vi "cp.vi"(5 "DLLPath":path, 6 "error in (no error)":errorcluster, 7 "CP Parameters":T2={"Steps"=[{"vs_initial"=FALSE, "Current_step"=0.0, "Duration_step"=1.0}, {"vs_initial"=FALSE, "Current_step"=0.001, "Duration_step"=1.0}, {"vs_initial"=FALSE, "Current_step"=0.005, "Duration_step"=1.0}], "Step_number"=2, "N_Cycles"=0, "Record_every_dE"=0.005, "Record_every_dT"=0.05, "I_Range"=8, "E_Range"=3, "Bandwidth"=5, "em"=1, "ce"=0, "tb"=2.5e-05} {"tb" min=2.5e-05 max=1 format="%^_3e"; "ce" items=["Standard", "CE to ground"]; "N_Cycles" min=0 max=1000000; "Step_number" min=0 max=99; "E_Range" items=["±2.5V", "±5V", "±10V", "Auto"]; "Bandwidth" items=["1"=1, "2"=2, "3"=3, "4"=4, "5"=5, "6"=6, "7"=7, "8"=8, "9"=9]; "Record_every_dT" min=0.0001 max=1000 format="%^_3e"; "Record_every_dE" format="%^_3e"; "I_Range" items=["1pA", "1nA", "10nA", "100nA", "1µA", "10µA", "100µA", "1mA", "10mA", "100mA", "1A", "Booster"]; "Steps"."Duration_step" min=0.001 max=80000 format="%^_3e"; "Steps"."Current_step" min=-150 max=150 format="%^_3e"}, 8 "Channel":u8(ring) items=["1", "2", "3", "4", "5", "6", "7", "8", "9", "10", "11", "12", "13", "14", "15", "16"], 9 "IP adress":string="192.109.209.229") -> (0 "error out":errorcluster, 1 "XY Graph":cluster{"Data 101":sgl[], "Data 101":sgl[]}(graph), 2 "output cluster":T1, 3 "Exit 2":bool=TRUE)   [LabVIEW 2022 SP3]
doc: "The Chrono-Potentiometry (CP) is a controlled current technique. The current is controlled and the potential is the variable determined as a function of time.\nIn general, in this VI, the first thing to do is to start by establishing the connection with the instrument defined by its IP adress, then load the firmware in the channel selected, get the information on the plugged channels, load protocol on a channel, start/stop the protocol, retreive data and draw the graph."
uses:
  Library/EClib Functions/CPParameters.ctl
  Library/EClib Functions/Parameters.ctl
  Library/EClib Functions/EClib functions.lvlib
panel:
  out "cycle index":i32[](array[numeric])
  in  "Display Parameters?":bool caption="Display Parameters"
  out "DllPath":path caption="DLL Path"
  out "LibVersion":string caption="DLL Version"
  in  "Draw":enum16{"Ewe(t)", "I(t)"}(ring)
  out "Number of points":i32=5992
  out "Data 102":sgl[][](array[numeric]) format="%.2f"
  in  "stop":bool
  in  "Exit":bool
  in  "Start":bool
  # "Instructions:\nBefore running the VI you must type a valid IP adress that corresponds to the instrument.Then press the Run button to execute this VI.\nWhile this VI is running, choose the available channel, enter the CP parameters or keep the default values, then press the start button to begin the experience.\nChoose the waveform to draw (Ewe(t) or I(t)). You can stop the measure if you press the stop button and exit the execution if you press the exit button."
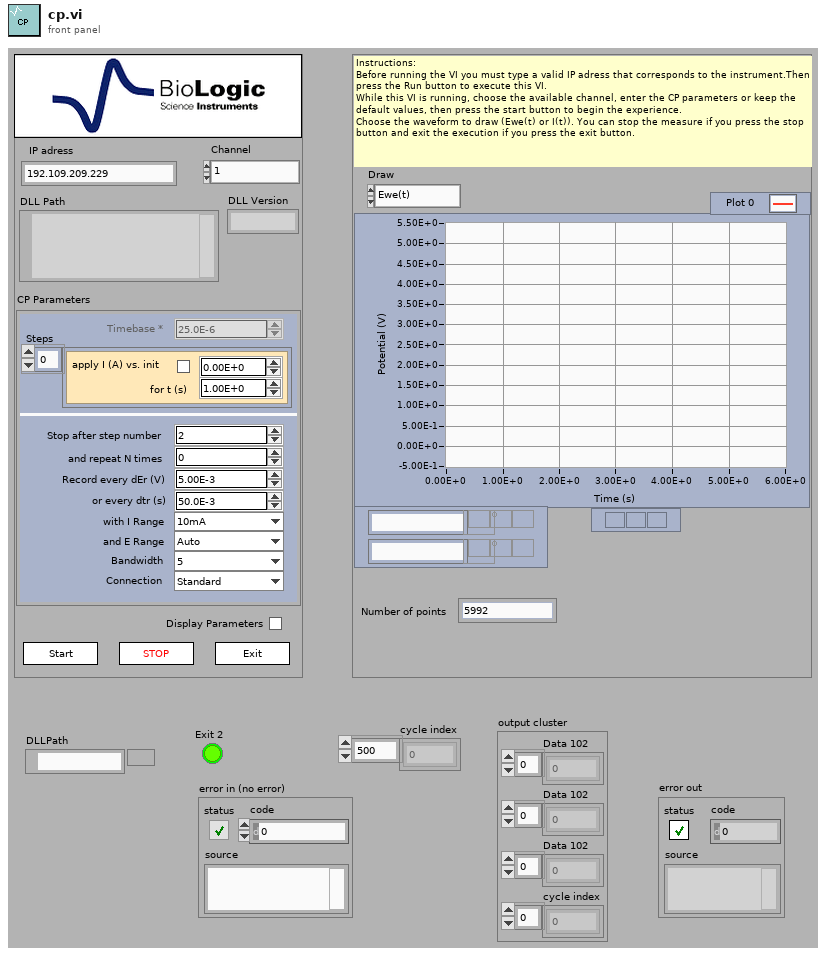
[diagram p1: front panel]
types:
  T1 = cluster{"Data 102":sgl[], "Data 102":sgl[], "Data 102":sgl[], "cycle index":i32[]}
  T2 = typedef "EClib functions.lvlib/CPParameters.ctl" = cluster{"Steps":cluster{"vs_initial":bool, "Current_step":sgl, "Duration_step":sgl}[], "Step_number":i32, "N_Cycles":i32, "Record_every_dE":sgl, "Record_every_dT":sgl, "I_Range":u16, "E_Range":u16, "Bandwidth":u16, "em":u16, "ce":u16, "tb":sgl}
  T3 = cluster{"LibVersion":string, "StringLength":u32, "DllPath":path}
  T4 = cluster{"Channel":i32, "BoardVersion":i32, "BoardSerialCode":i32, "FirmwareCode":i32, "FirmwareVersion":i32, "XilinxVersion":i32, "AmpCode":i32, "NbAmp":i32, "LcBoard":i32, "Zboard":i32, "MuxBoard":i32, "GPRAboard":i32, "MemSize":i32, "MemFilled":i32, "state":i32, "MaxIRange":i32, "MinIRange":i32, "MaxBandwidth":i32, "NbOfTechniques":i32}
  T5 = typedef "EClib functions.lvlib/Parameters.ctl" = enum16{"CA", "CASG", "CP", "GEIS", "ISCAN", "OCV", "PEIS", "SCCX", "SGEIS", "SPEIS", "VSCAN", "MP"}
  T6 = typedef "EClib functions.lvlib/TechniqueParameters.ctl" = cluster{"String Label":string, "Type":i32, "Valeur":i32, "Index":i32}
  T7 = cluster{"string before end tag":string, i32, i32, i32}[]
  T8 = cluster{"IRQskipped":i32, "NbRaws":i32, "NbCols":i32, "Technique Index":i32, "TechniqueID":i32, "PrcessIndex":i32, "loop":i32, "StartTime":dbl, "MuxPad":i32}
  T9 = cluster{"State":i32, "MemFilled":i32, "TimeBase":sgl, " Ewe":sgl, " EweRangeMin":sgl, " EweRangeMax":sgl, "Ece":sgl, "EceRangeMin":sgl, "EceRangeMax":sgl, "Eoverflow":i32, "I":sgl, "IRange":i32, "Ioverflow":i32, "ElapsedTime":sgl, "Freq":sgl, "Rcomp":sgl, "Saturation":sgl, "OptErr":i32, "OptPos":i32}
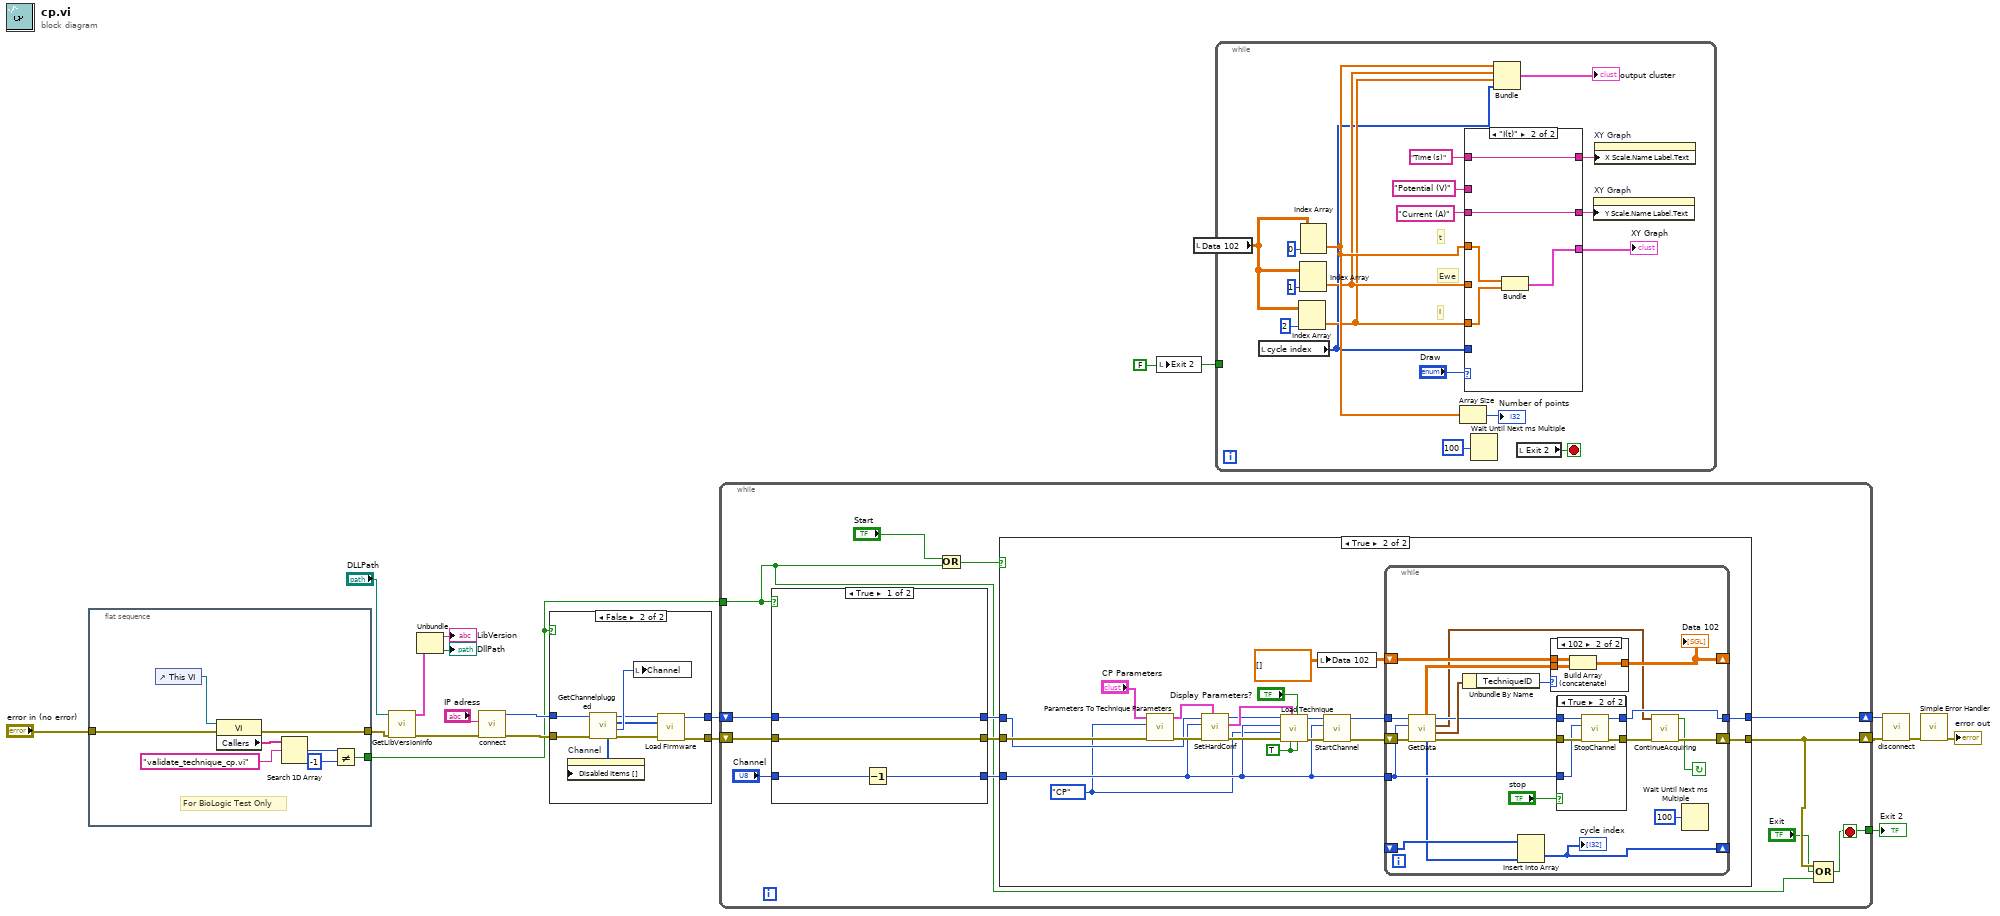
[diagram p0: block diagram]
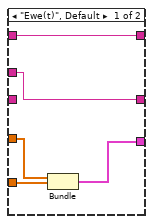
[diagram p3: hidden frame]
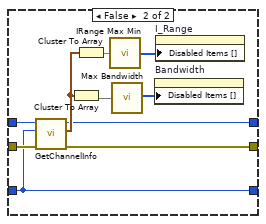
[diagram p4: hidden frame]
diagram:
  w18 = FALSE ("Exit 2")
  n1 = flat-sequence {
    tunnel: "error in (no error)" -> [w26]
    tunnel: [w25] -> w5
    tunnel: [w20] -> w3
    frame #0 {
      # "For BioLogic Test Only"
      n2 = control-ref of="This VI"() -> (w27:refnum<vi>)
      n3 = property class="VI"(reference=w27, error in=w26) -> (error out=w25:errorcluster, "Callers"=w24:string[])  [unwired: 1 out]
      n4 = Search 1D Array(1D array=w24, element="validate_technique_cp.vi") -> (index of element=w22:i32)  [unwired: 1 in]
      n5 = Not Equal?(x=w22, y=-1) -> (x != y?=w20:bool)
    }
  }
  n6 = call "GetLibVersionInfo.vi"("error in (no error)"=w5, "DLLPath"="DLLPath") -> ("error out"=w6:errorcluster, "LibInfo"=w9:T3)  [unwired: 8 in]
  n7 = Unbundle(w9) -> ("LibVersion"=→"LibVersion":string, "DllPath"=→"DllPath":path)  [unwired: 1 out]
  n8 = call "connect.vi"("error in (no error)"=w6, "IP"="IP adress") -> ("error out"=w15:errorcluster, "ID Out"=w13:i32)  [unwired: 5 in, 3 out]
  n9 = case shown="False" w3 {
    tunnel: w15 -> [w28 w37]
    tunnel: [w28 w35] -> w14
    tunnel: w13 -> [w29 w33]
    tunnel: [w29 w32] -> w12
    frame True {
    }
    frame False {
      n10 = call "GetChannelplugged.vi"("error in (no error)"=w37, "ID In"=w33) -> ("error out"=w36:errorcluster, "FirstPluggedChannel"=w38:u8, "PluggedChannels"=w30:u8[], "ID Out"=w34:i32, "DisabledChannels"=w31:i32[])  [unwired: 5 in]
      n11 = property on="Channel" class="Ring (strict)"("Disabled Items []"=w31) -> ()  [unwired: 2 in, 2 out]
      n12 = local write "Channel"(w38) -> ()
      n13 = call "Load Firmware.vi"("error in (no error)"=w36, "Channels"=w30, "ID In"=w34) -> ("error out"=w35:errorcluster, "ID Out"=w32:i32)  [unwired: 6 in, 1 out]
    }
  }
  n14 = while {
    shift-right: [w42] -> w11
    shift-left: w14 -> [w50]
    tunnel: [w39] -> w19
    shift-right: [w51] -> w16
    shift-left: w12 -> [w47]
    tunnel: w3 -> [w40]
    stop <- w39 stop-if-true
    n15 = case shown="True" w40 {
      tunnel: w50 -> [w52 w61]
      tunnel: "Channel" -> [w54 w56]
      tunnel: [w52 w60] -> w48
      tunnel: w47 -> [w55 w58]
      tunnel: [w55 w57] -> w46
      tunnel: [w53 w56] -> w45
      frame True {
        n16 = Decrement(x=w54) -> (x-1=w53:u8)
      }
      frame False {
        n17 = call "GetChannelInfo.vi"("error in (no error)"=w61, "Channel"=w56, "ID"=w58) -> ("error out"=w60:errorcluster, "Channel information"=w59:T4, "ID Out"=w57:i32)  [unwired: 6 in]
        n18 = Cluster To Array(cluster=w59) -> (array=w64:i32[])
        n19 = Cluster To Array(cluster=w59) -> (array=w65:i32[])
        n20 = call "IRange Max Min.vi"("resources"=w65) -> ("disabled ranges"=w63:i32[])
        n21 = call "Max Bandwidth.vi"("resources"=w64) -> ("disabled ranges"=w62:i32[])
        n22 = property on="Bandwidth" class="Ring (strict)"("Disabled Items []"=w62) -> ()  [unwired: 2 in, 2 out]
        n23 = property on="I_Range" class="Ring (strict)"("Disabled Items []"=w63) -> ()  [unwired: 2 in, 2 out]
      }
    }
    n24 = Or(x="Start", y=w40) -> (x .or. y?=w43:bool)
    n25 = case shown="True" w43 {
      tunnel: w45 -> [_ w70]
      tunnel: [w67 w86] -> w42
      tunnel: w48 -> [w67 w71]
      tunnel: w46 -> [w66 w69]
      tunnel: [w66 w78] -> w51
      frame False {
      }
      frame True {
        w68 = Parameters."CP" ("Parameters")
        w79 = TRUE ("First Protocol")
        w85 = sgl[][] []
        n26 = call "Parameters To Technique Parameters.vi"("error in (no error)"=w71, "Parameters"=w68, "ParameterIN"="CP Parameters") -> ("error out"=w77:errorcluster, "Params Values"=w76:T6[])  [unwired: 7 in]
        n27 = call "SetHardConf.vi"("Params Values"=w76, "error in (no error)"=w77, "Channel"=w70, "ID In"=w69) -> ("error out"=w73:errorcluster, "Params Values Trimed"=w75:T7, "ID Out"=w74:i32)  [unwired: 5 in]
        n28 = call "Load Technique.vi"("Last Protocol"=w79, "Display Parameters?"="Display Parameters?", "First Protocol"=w79, "TechniqueParameters"=w75, "error in (no error)"=w73, "Parameters"=w68, "Selected Channel"=w70, "ID In"=w74) -> ("error out"=w82:errorcluster, "ID  Out"=w81:i32)  [unwired: 1 in, 1 out]
        n29 = local write "Data 102"(w85) -> ()
        n30 = call "StartChannel.vi"("error in (no error)"=w82, "Channel"=w70, "ID In"=w81) -> ("error out"=w83:errorcluster, "ID Out"=w80:i32)  [unwired: 7 in]
        n31 = while {
          shift-right: [w93] -> w86
          shift-left: w83 -> [w106]
          shift-right: [w103] -> _
          shift-left: w85 -> [w104]
          tunnel: w70 -> [w95]
          tunnel: w80 -> [w101]
          tunnel: [w96] -> w78
          shift-right: [w89] -> _
          shift-left: _ -> [w88]
          stop <- w91 continue-if-true
          n32 = call "GetData.vi"("error in (no error)"=w106, "Channel"=w95, "ID In"=w101) -> ("error out"=w94:errorcluster, "Data information"=w100:T8, "Current values"=w90:T9, "ID Out"=w97:i32, "row2"=w87:u32[], "Data"=w98:dbl[][])  [unwired: 1 in, 2 out]
          n33 = Unbundle By Name(w100) -> ("TechniqueID"=w99:i32)
          n34 = Insert Into Array(array=w88, new element=w87) -> (w89:u32[])  [unwired: 1 in]
          "cycle index" <- w89
          n35 = case shown="102" w99 {
            tunnel: w98 -> [_ w117]
            tunnel: w104 -> [w114 w116]
            tunnel: [w114 w115] -> w103
            frame 0, Default {
            }
            frame 102 {
              n36 = Build Array (concatenate)(w116, w117) -> (w115:dbl[][])
            }
          }
          "Data 102" <- w103
          n37 = case shown="True" "stop" {
            tunnel: [w108 w113] -> w92
            tunnel: w94 -> [w108 w112]
            tunnel: w97 -> [w107 w111]
            tunnel: [w107 w110] -> w96
            tunnel: w95 -> [_ w109]
            frame False {
            }
            frame True {
              n38 = call "StopChannel.vi"("error in (no error)"=w112, "Channel"=w109, "ID In"=w111) -> ("error out"=w113:errorcluster, "ID Out"=w110:i32)  [unwired: 7 in]
            }
          }
          n39 = call "ContinueAcquiring.vi"("error in"=w92, "Current values"=w90) -> ("error out"=w93:errorcluster, "ContinueAcquiring?"=w91:bool)  [unwired: 8 in]
          n40 = Wait Until Next ms Multiple(millisecond multiple=u32 100) -> ()  [unwired: 1 out]
        }
      }
    }
    n41 = Compound Arithmetic op=OR(w42, "Exit", w40) -> (w39:bool)
  }
  "Exit 2" <- w19
  n42 = local write "Exit 2"(w18) -> ()
  n43 = while {
    tunnel: w18 -> [_]
    stop <- w135 stop-if-true
    # "I"
    # "Ewe"
    # "t"
    n44 = local read "Data 102"() -> (w124:sgl[][])
    n45 = local read "cycle index"() -> (w119:i32[])
    n46 = Index Array(array=w124, index (col)=2 ("indice désactivé (col)")) -> (element=w120:sgl[])  [unwired: 1 in]
    n47 = Index Array(array=w124, index (col)=1 ("Index")) -> (element=w121:sgl[])  [unwired: 1 in]
    n48 = Index Array(array=w124, index (col)=0 ("Index")) -> (element=w122:sgl[])  [unwired: 1 in]
    n49 = Array Size(array=w122) -> (size(s)=→"Number of points":i32)
    n50 = case shown="\"I(t)\"" "Draw" {
      tunnel: w122 -> [w141 w146]
      tunnel: [w138 w142] -> w123
      tunnel: "Potential (V)" ("Y Scale.Name Label.Text") -> [w140 _]
      tunnel: "Current (A)" ("Y Scale.Name Label.Text") -> [_ w145]
      tunnel: [w140 w145] -> w129
      tunnel: [w139 w144] -> w128
      tunnel: "Time (s)" ("Y Scale.Name Label.Text") -> [w139 w144]
      tunnel: w121 -> [w137 _]
      tunnel: w120 -> [_ w143]
      tunnel: w119 -> [_ _]
      frame "Ewe(t)", Default {
        n51 = Bundle("Data 102"=w141, "Data 102"=w137) -> (w138:cluster{"Data 102":sgl[], "Data 102":sgl[]})  [unwired: 1 in]
      }
      frame "I(t)" {
        n52 = Bundle("Data 102"=w146, "Data 102"=w143) -> (w142:cluster{"Data 102":sgl[], "Data 102":sgl[]})  [unwired: 1 in]
      }
    }
    "XY Graph" <- w123
    n53 = Wait Until Next ms Multiple(millisecond multiple=u32 100) -> ()  [unwired: 1 out]
    n54 = Bundle("Data 102"=w122, "Data 102"=w121, "Data 102"=w120, "cycle index"=w119) -> (→"output cluster":T1)  [unwired: 1 in]
    n55 = local read "Exit 2"() -> (w135:bool)
    n56 = property on="XY Graph" class="XYGraph (strict)"("Y Scale.Name Label.Text"=w129) -> ()  [unwired: 2 in, 2 out]
    n57 = property on="XY Graph" class="XYGraph (strict)"("X Scale.Name Label.Text"=w128) -> ()  [unwired: 2 in, 2 out]
  }
  n58 = call "disconnect.vi"("error in (no error)"=w11, "ID In"=w16) -> ("error out"=w10:errorcluster)  [unwired: 9 in]
  n59 = call <vilib>:"Simple Error Handler.vi"("error in (no error)"=w10) -> ("error out"=→"error out":errorcluster)  [unwired: 4 in, 4 out]
